vi "zmq_ctx_check.vi"(1 "context in":refnum<class "zmq_context.lvclass">) -> (0 "valid?":bool)   [LabVIEW 2019, in "zeromq.lvlib" / "zmq_context.lvclass"]
doc: "Checks whether the supplied context object is valid"
uses:
  zmq_context.lvclass
  zmq_context.lvclass/zmq_context.ctl
  zeromq.lvlib
panel:
  # "ØMQ"
  # "labview"
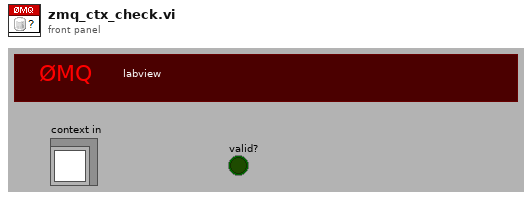
[diagram p1: front panel]
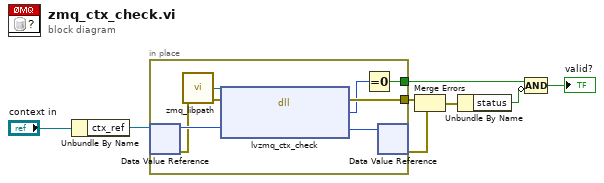
[diagram p0: block diagram]
diagram:
  n1 = Unbundle By Name("context in") -> ("ctx_ref"=w7:refnum<data-value>)
  n2 = in-place {
    in-place-border: [w11] -> w6
    in-place-border: [w9] -> w3
    n3 = in-place-dvr #1(w7) -> (w15:u64, w12:errorcluster)
    n4 = call "zmq_libpath.vi"() -> ("path"=w13:path)
    n5 = dll-call lib="?" fn="lvzmq_ctx_check" ("zmq_labview.dll:lvzmq_socket")(path in=w13, error in=w12, "ctx_obj"=w15) -> (error out=w11:errorcluster, "return type"=w10:i32, "ctx_obj"=w14:u64)  [unwired: 1 in, 1 out]
    n6 = Equal To 0?(x=w10) -> (x = 0?=w9:bool)
    n7 = in-place-dvr #1(w14) -> (w5:errorcluster)  [unwired: 1 out]
  }
  n8 = Merge Errors(w6, w5) -> (w4:errorcluster)
  n9 = Unbundle By Name(w4) -> ("status"=w2:bool)
  n10 = Compound Arithmetic op=AND(w3, invert w2) -> (→"valid?":bool)
